vi "BM Empty Filters.vi"(8 "error in (no error)":errorcluster, 11 "Bus Monitor in":refnum<class "Bus Monitor.lvclass">) -> (0 "error out":errorcluster, 3 "Bus Monitor out":refnum<class "Bus Monitor.lvclass">)   [LabVIEW 2020, in "Unit Tests.lvlib" / "Bus Monitor.lvclass"]
uses:
  Bus Monitor.lvclass
  Bus Monitor.lvclass/Bus Monitor.ctl
  <vilib>/addons/_JKI Toolkits/Caraya/classes/Assert/Assert True.vi
  Dependencies/FPGA Interface/FPGA Interface.lvclass
  <vilib>/addons/_JKI Toolkits/Caraya/classes/Test/Test.lvclass
  <vilib>/addons/_JKI Toolkits/Caraya/classes/Assert/Assert.lvclass
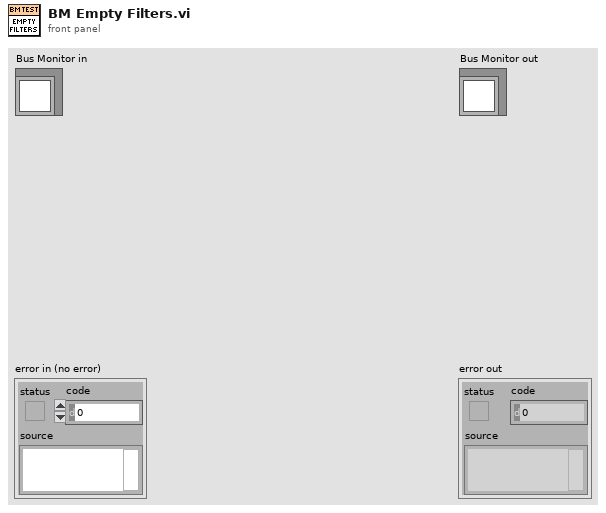
[diagram p1: front panel]
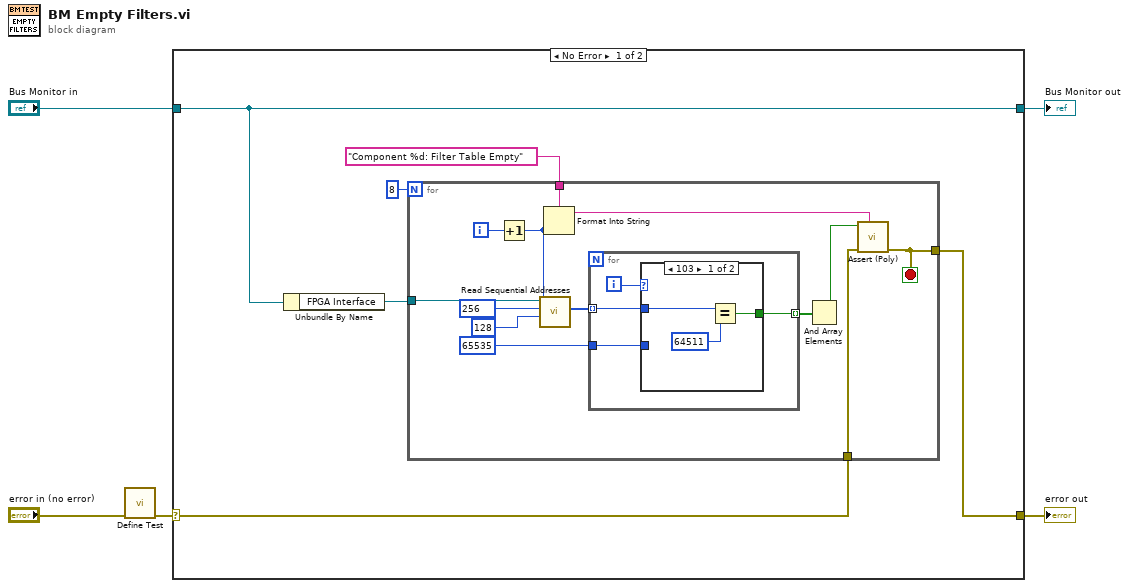
[diagram p0: block diagram]
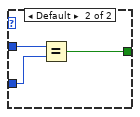
[diagram p2: hidden frame]
diagram:
  n1 = call <vilib>:"Define Test.vi"("error in (no error)"="error in (no error)") -> ("error out"=w1:errorcluster)  [unwired: 9 in, 1 out]
  n2 = case shown="No Error" w1 {
    selector: w1 -> [w9 w36]
    tunnel: [w8 w36] -> w5
    tunnel: [w11 w35] -> w3
    tunnel: "Bus Monitor in" -> [w11 w35]
    frame No Error {
      n3 = Unbundle By Name(w11) -> ("FPGA Interface"=w10:refnum<class "FPGA Interface.lvclass">)
      n4 = for {
        N: 8 -> [_]
        tunnel: "Component %d: Filter Table Empty" ("custom report message (\"\")") -> [w23]
        tunnel: w9 -> [w13]
        tunnel: [w14] -> w8
        tunnel: w10 -> [w22]
        i -> [w24]
        stop <- w14 stop-if-true
        n5 = Increment(x=w24) -> (x+1=w21:i32)
        n6 = call-dynamic "Read Sequential Addresses.vi"("Target IC (1-8)"=w21, "Addresses to Read"=u16 128, "Starting Address"=u16 256, "FPGA Interface in"=w22) -> ("Data"=w18:u16[])  [unwired: 6 in, 1 out]
        n7 = Format Into String(format string=w23, w21) -> (resulting string=w12:string)  [unwired: 2 in, 1 out]
        n8 = for {
          tunnel: w18 -> [w27] mode=indexing
          tunnel: u16 65535 -> [w26]
          tunnel: [w25] -> w16 mode=indexing
          i -> [w28]
          n9 = case shown="103" w28 {
            tunnel: w27 -> [w31 w34]
            tunnel: w26 -> [_ w33]
            tunnel: [w30 w32] -> w25
            frame 103 {
              n10 = Equal?(x=w31, y=u16 64511) -> (x = y?=w30:bool)
            }
            frame Default {
              n11 = Equal?(x=w34, y=w33) -> (x = y?=w32:bool)
            }
          }
        }
        n12 = And Array Elements(Boolean array=w16) -> (logical AND=w15:bool)
        n13 = call-poly <vilib>:"Assert (Poly).vi"("Label"=w12, "error in (no error)"=w13, "True?"=w15) -> ("error out"=w14:errorcluster)  [unwired: 7 in, 1 out]
      }
    }
    frame Error {
    }
  }
  "error out" <- w5
  "Bus Monitor out" <- w3
